vi "Process and save image.vi"(0 "Refnum in":T2, 1 "New Image":T1, 7 "Numeric":i32, 11 "error in (no error)":errorcluster) -> (4 "Refnum out":T1, 6 "logfile name":path, 8 "Particle Measurements (Pixels)":dbl[][](array[numeric]), 15 "error out":errorcluster)   [LabVIEW 2019]
uses:
  <vilib>/vision/Image Controls.llb/IMAQ Image.ctl
  <vilib>/userDefined/High Color/IMAQdx.ctl
  <vilib>/vision/driver/NI_Vision_Acquisition_Software.lvlib
  <vilib>/vision/NI_Vision_Development_Module.lvlib
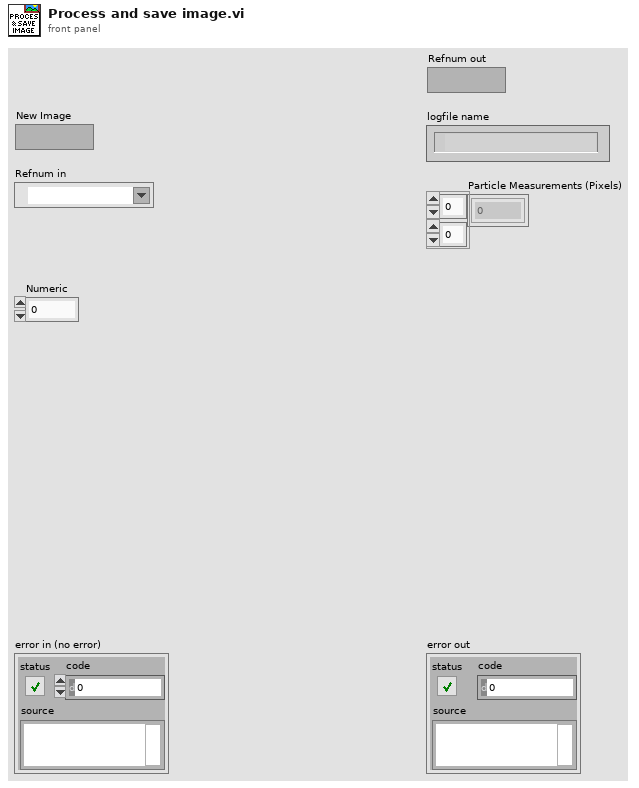
[diagram p1: front panel]
types:
  T1 = typedef "IMAQ Image.ctl" = refnum<image>
  T2 = typedef "IMAQdx.ctl" = refnum<k21>
  T3 = enum32{"AutoM", "Close", "Dilate", "Erode", "Gradient", "Gradient out", "Gradient in", "Hit miss", "Open", "PClose", "POpen", "Thick", "Thin"}
  T4 = typedef "Image Type" = u32
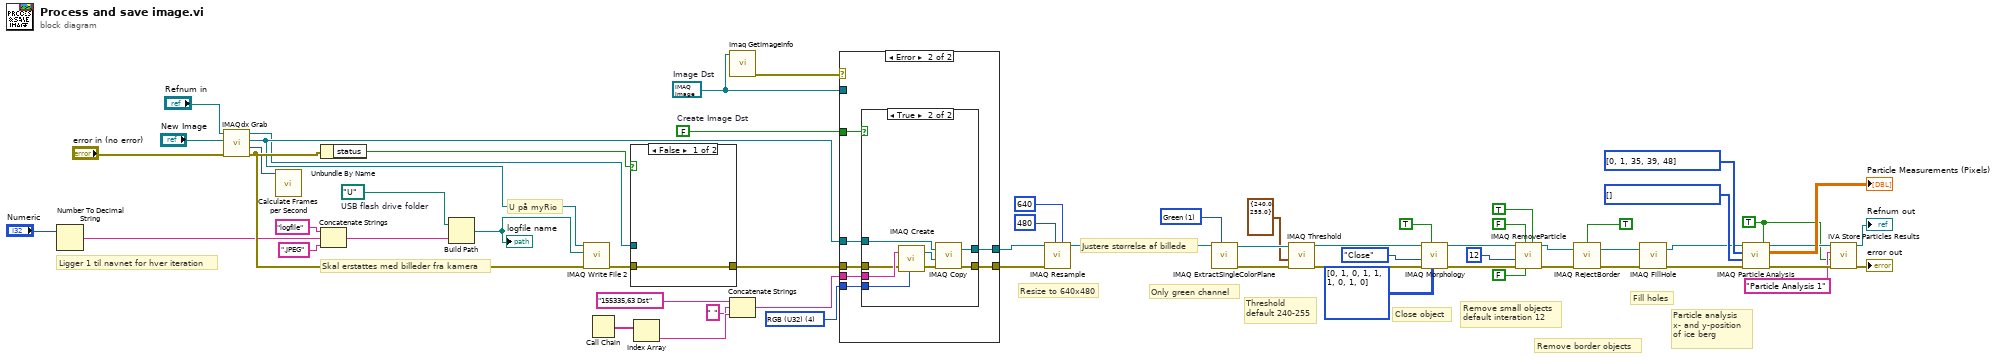
[diagram p0: block diagram]
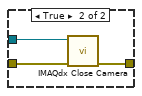
[diagram p2: hidden frame]
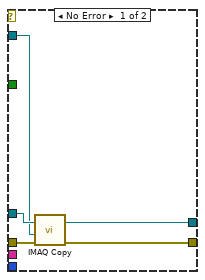
[diagram p3: hidden frame]
diagram:
  w31 = 1 items=["Red", "Green", "Blue", "Hue", "Saturation", "Luminance", "Value", "Intensity"] ("Color Plane (Color Plane Extraction 1)")
  w50 = i32[] [] items=["Center of Mass X", "Center of Mass Y", "First Pixel X", "First Pixel Y", "Bounding Rect Left", "Bounding Rect Top", "Bounding Rect Right", "Bounding Rect Bottom", "Max Feret Diameter Start X", "Max Feret Diameter Start Y", "Max Feret Diameter End X", "Max Feret Diameter End Y", "Max Horiz. Segment Length Left", "Max Horiz. Segment Length Right", "Max Horiz. Segment Length Row", "-", "Bounding Rect Width", "Bounding Rect Height", "Bounding Rect Diagonal", "Perimeter", "Convex Hull Perimeter", "Holes' Perimeter", "Max Feret Diameter", "Equivalent Ellipse Major Axis", "Equivalent Ellipse Minor Axis", "Equivalent Ellipse Minor Axis (Feret)", "Equivalent Rect Long Side", "Equivalent Rect Short Side", "Equivalent Rect Diagonal", "Equivalent Rect Short Side (Feret)", "Average Horiz. Segment Length", "Average Vert. Segment Length", "Hydraulic Radius", "Waddel Disk Diameter", "-", "Area", "Holes' Area", "Particle & Holes' Area", "Convex Hull Area", "Image Area", "-", "Number of Holes", "Number of Horiz. Segments", "Number of Vert. Segments", "-", "Orientation", "Max Feret Diameter Orientation", "-", "% Area/Image Area", "% Area/(Particle & Holes' Area)", "Ratio of Equivalent Ellipse Axes", "Ratio of Equivalent Rect Sides", "-", "Elongation Factor", "Compactness Factor", "Heywood Circularity Factor", "Type Factor", "-", "Sum X", "Sum Y", "Sum XX", "Sum XY", "Sum YY", "Sum XXX", "Sum XXY", "Sum XYY", "Sum YYY", "-", "Moment of Inertia XX", "Moment of Inertia XY", "Moment of Inertia YY", "Moment of Inertia XXX", "Moment of Inertia XXY", "Moment of Inertia XYY", "Moment of Inertia YYY", "Norm. Moment of Inertia XX", "Norm. Moment of Inertia XY", "Norm. Moment of Inertia YY", "Norm. Moment of Inertia XXX", "Norm. Moment of Inertia XXY", "Norm. Moment of Inertia XYY", "Norm. Moment of Inertia YYY", "Hu Moment 1", "Hu Moment 2", "Hu Moment 3", "Hu Moment 4", "Hu Moment 5", "Hu Moment 6", "Hu Moment 7"] ("Real-World Measurements")
  w49 = i32[] [0, 1, 35, 39, 48] items=["Center of Mass X", "Center of Mass Y", "First Pixel X", "First Pixel Y", "Bounding Rect Left", "Bounding Rect Top", "Bounding Rect Right", "Bounding Rect Bottom", "Max Feret Diameter Start X", "Max Feret Diameter Start Y", "Max Feret Diameter End X", "Max Feret Diameter End Y", "Max Horiz. Segment Length Left", "Max Horiz. Segment Length Right", "Max Horiz. Segment Length Row", "-", "Bounding Rect Width", "Bounding Rect Height", "Bounding Rect Diagonal", "Perimeter", "Convex Hull Perimeter", "Holes' Perimeter", "Max Feret Diameter", "Equivalent Ellipse Major Axis", "Equivalent Ellipse Minor Axis", "Equivalent Ellipse Minor Axis (Feret)", "Equivalent Rect Long Side", "Equivalent Rect Short Side", "Equivalent Rect Diagonal", "Equivalent Rect Short Side (Feret)", "Average Horiz. Segment Length", "Average Vert. Segment Length", "Hydraulic Radius", "Waddel Disk Diameter", "-", "Area", "Holes' Area", "Particle & Holes' Area", "Convex Hull Area", "Image Area", "-", "Number of Holes", "Number of Horiz. Segments", "Number of Vert. Segments", "-", "Orientation", "Max Feret Diameter Orientation", "-", "% Area/Image Area", "% Area/(Particle & Holes' Area)", "Ratio of Equivalent Ellipse Axes", "Ratio of Equivalent Rect Sides", "-", "Elongation Factor", "Compactness Factor", "Heywood Circularity Factor", "Type Factor", "-", "Sum X", "Sum Y", "Sum XX", "Sum XY", "Sum YY", "Sum XXX", "Sum XXY", "Sum XYY", "Sum YYY", "-", "Moment of Inertia XX", "Moment of Inertia XY", "Moment of Inertia YY", "Moment of Inertia XXX", "Moment of Inertia XXY", "Moment of Inertia XYY", "Moment of Inertia YYY", "Norm. Moment of Inertia XX", "Norm. Moment of Inertia XY", "Norm. Moment of Inertia YY", "Norm. Moment of Inertia XXX", "Norm. Moment of Inertia XXY", "Norm. Moment of Inertia XYY", "Norm. Moment of Inertia YYY", "Hu Moment 1", "Hu Moment 2", "Hu Moment 3", "Hu Moment 4", "Hu Moment 5", "Hu Moment 6", "Hu Moment 7"] ("Pixel Measurements")
  w51 = TRUE ("Connectivity 4/8 (8)")
  w30 = path "U:/"  # USB flash drive folder
  w5 = T1 refnum  # Image Dst
  w13 = T4 4 items=["Grayscale (U8)", "Grayscale (I16)", "Grayscale (SGL)", "Complex (CSG)", "RGB (U32)", "HSL (U32)", "RGB (U64)", "Grayscale (U16)"] ("Image Dst Type")
  w7 = FALSE  # Create Image Dst
  # "Particle analysis\nx- and y-position\nof ice berg"
  # "Fill holes"
  # "Remove border objects"
  # "Remove small objects\ndefault interation 12"
  # "Close object"
  # "Threshold\ndefault 240-255"
  # "Only green channel"
  # "Resize to 640x480"
  # "Justere størrelse af billede"
  # "U på myRio"
  # "Ligger 1 til navnet for hver iteration"
  # "Skal erstattes med billeder fra kamera"
  n1 = Number To Decimal String(number="Numeric") -> (decimal integer string=w24:string)  [unwired: 1 in]
  n2 = call <vilib>:"IMAQdx Grab.vi"("error in"="error in (no error)", "Image In"="New Image", "Session In"="Refnum in") -> ("error out"=w27:errorcluster, "Buffer Number Out"=w15:u32, "Image Out"=w26:T1, "Session Out"=w16:T2)  [unwired: 1 in, 4 out]
  n3 = call <vilib>:"Calculate Frames per Second.vi"("Buffer Number"=w15) -> ()  [unwired: 2 in, 9 out]
  n4 = Unbundle By Name(w27) -> ("status"=w20:bool)
  n5 = Concatenate Strings "Concatenate Strings"("logfile" ("logfile base name"), w24, ".JPEG" ("string")) -> (w22:string)
  n6 = Build Path(base path=w30, name or relative path=w22) -> (appended path=w21:path)
  "logfile name" <- w21
  n7 = call-poly "IMAQ Write File 2"("error in (no error)"=w27, "File Path"=w21, "Image"=w26) -> ("error out"=w28:errorcluster)  [unwired: 7 in, 1 out]
  n8 = Call Chain() -> (call chain=w8:string[])
  n9 = case "Case Structure_template1" shown="False" w20 {
    tunnel: [w63 w65] -> w17
    tunnel: w28 -> [w63 w66]
    tunnel: w16 -> [_ w64]
    frame False {
    }
    frame True {
      n10 = call <vilib>:"IMAQdx Close Camera.vi"("error in"=w66, "Session In"=w64) -> ("error out"=w65:errorcluster)  [unwired: 9 out]
    }
  }
  n11 = Index Array(array=w8) -> (element=w10:string)  [unwired: 1 in]
  n12 = call "Imaq GetImageInfo"("Image"=w5) -> ("error out"=w6:errorcluster)  [unwired: 1 in, 9 out]
  n13 = Concatenate Strings("155335,63 Dst" ("Image Dst Name"), " ", w10) -> (w12:string)
  n14 = case shown="Error" w6 {
    tunnel: [w71 w75] -> w57
    tunnel: [w70 w74] -> w58
    tunnel: w26 -> [w69 w76]
    tunnel: w17 -> [w68 w72]
    tunnel: w5 -> [w67 _]
    tunnel: w12 -> [_ w78]
    tunnel: w13 -> [_ w77]
    tunnel: w7 -> [_ w73]
    frame No Error {
      n15 = call "IMAQ Copy"("error in (no error)"=w68, "Image Dst"=w67, "Image Src"=w69) -> ("error out"=w70:errorcluster, "Image Dst Out"=w71:T1)  [unwired: 3 out]
    }
    frame Error {
      n16 = case shown="True" w73 {
        tunnel: w78 -> [_ w88]
        tunnel: w77 -> [_ w87]
        tunnel: w76 -> [w80 w85]
        tunnel: [w80 w84] -> w75
        tunnel: [w79 w83] -> w74
        tunnel: w72 -> [w79 w81]
        frame False {
        }
        frame True {
          n17 = call "IMAQ Create"("Image Name"=w88, "Image Type"=w87, "error in (no error)"=w81) -> ("New Image"=w86:T1, "error out"=w82:errorcluster)  [unwired: 1 in, 1 out]
          n18 = call "IMAQ Copy"("error in (no error)"=w82, "Image Dst"=w86, "Image Src"=w85) -> ("error out"=w83:errorcluster, "Image Dst Out"=w84:T1)  [unwired: 3 out]
        }
      }
    }
  }
  n19 = call "IMAQ Resample"("X Resolution"=u16 640 ("Width"), "Y Resolution"=u16 480 ("Height"), "error in (no error)"=w58, "Image Src"=w57) -> ("Image Dst Out"=w60:T1)  [unwired: 6 in, 1 out]
  n20 = call "IMAQ ExtractSingleColorPlane"("Color Plane"=w31, "Image Src"=w60) -> ("error out"=w32:errorcluster, "Image Dst Out"=w34:T1)  [unwired: 2 in, 6 out]
  n21 = call "IMAQ Threshold"("error in (no error)"=w32, "Range"=cluster{"Lower value":sgl, "Upper value":sgl} {"Lower value"=240.0, "Upper value"=255.0} ("Range (Threshold 1)"), "Image Src"=w34) -> ("error out"=w35:errorcluster, "Image Dst Out"=w39:T1)  [unwired: 3 in, 4 out]
  n22 = call "IMAQ Morphology"("Structuring Element"=i32[][] [[0, 1, 0], [1, 1, 1], [0, 1, 0]] ("Structuring Element (Basic Morphology 1)"), "Square/Hexa (Square)"=TRUE, "error in (no error)"=w35, "Operation"=T3."Close", "Image Src"=w39) -> ("error out"=w40:errorcluster, "Image Dst Out"=w45:T1)  [unwired: 2 in, 3 out]
  n23 = call "IMAQ RemoveParticle"("Connectivity 4/8 (8)"=TRUE, "Low Pass/High Pass (Low)"=FALSE, "Square/Hexa (Square)"=FALSE, "error in (no error)"=w40, "Number of Erosion"=12 ("Number of Erosion (Advanced Morphology 1)"), "Image Src"=w45) -> ("error out"=w46:errorcluster, "Image Dst Out"=w48:T1)  [unwired: 1 in, 3 out]
  n24 = call "IMAQ RejectBorder"("error in (no error)"=w46, "Image Src"=w48, "Connectivity 4/8 (8)"=TRUE) -> ("error out"=w1:errorcluster, "Image Dst Out"=w4:T1)  [unwired: 1 in, 2 out]
  n25 = call "IMAQ FillHole"("error in (no error)"=w1, "Image Src"=w4) -> ("error out"=w2:errorcluster, "Image Dst Out"=w3:T1)  [unwired: 4 in]
  n26 = call "IMAQ Particle Analysis"("Connectivity 4/8 (8)"=w51, "error in (no error)"=w2, "Real-World Measurements"=w50, "Pixel Measurements"=w49, "Image"=w3) -> ("error out"=w54:errorcluster, "Particle Measurements (Pixels)"=→"Particle Measurements (Pixels)":dbl[][], "Image Out (duplicate)"=w52:T1)  [unwired: 4 out]
  n27 = call <vilib>:"IVA Store Particles Results.vi"("error in (no error)"=w54, "Connectivity 4/8 (8)"=w51, "Step Name"="Particle Analysis 1", "Image in"=w52) -> ("error out"=→"error out":errorcluster, "Image dup"=→"Refnum out":T1)  [unwired: 6 out]
